vi "Get TargetRoot.vi"(8 "error in (no error)":errorcluster, 11 "Installation Directory":path) -> (0 "error out":errorcluster, 1 "Target Root Name":string, 2 "Relative Path":path)   [LabVIEW 2019, in "NIPKG Packager.lvclass"]
doc: "Calculates the Target Root directory for the NIPM Package. This is a fairly long list of potential root directories, but only a subset of common directories are handled here. This might mean in some circumstances the returned relative path is longer that if a larger collection of target roots were considered."
uses:
  NIPKG Packager.lvclass
  <vilib>/Utility/sysdir.llb/System Directory Type.ctl
  <vilib>/Utility/error.llb/Error Cluster From Error Code.vi
  <vilib>/ErrorRing/Error Ring.xnode
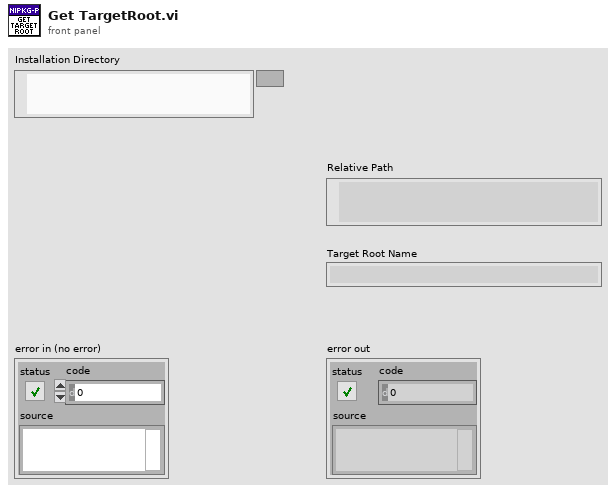
[diagram p1: front panel]
types:
  T1 = typedef "System Directory Type.ctl" = i32
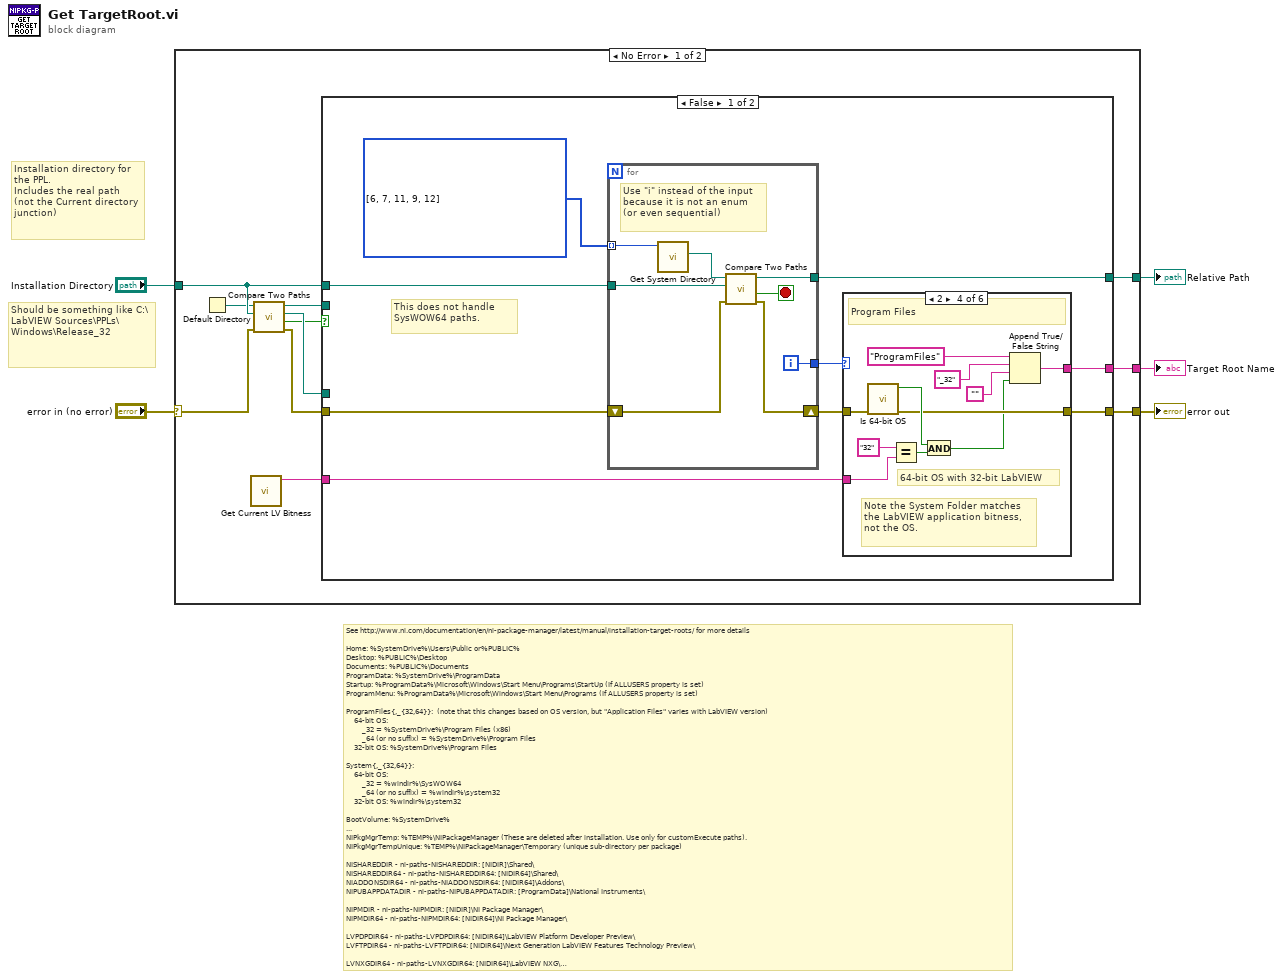
[diagram p0: block diagram]
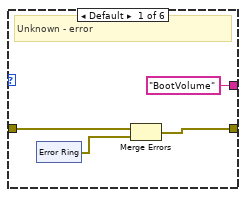
[diagram p2: hidden frame]
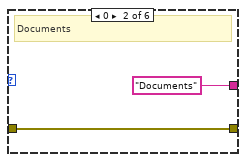
[diagram p3: hidden frame]
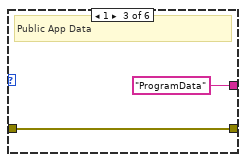
[diagram p4: hidden frame]
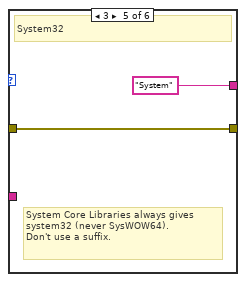
[diagram p5: hidden frame]
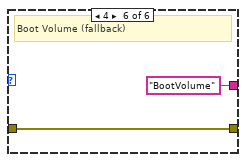
[diagram p6: hidden frame]
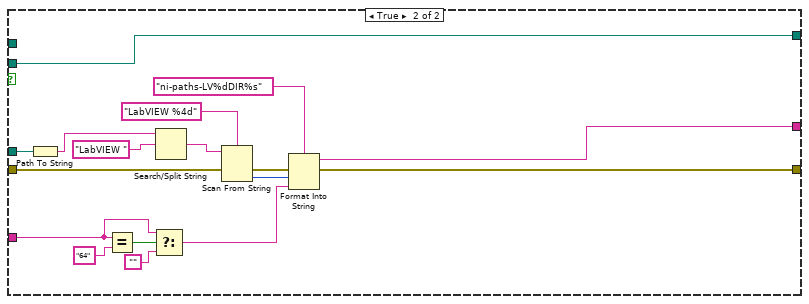
[diagram p7: hidden frame]
diagram:
  # "Should be something like C:\\LabVIEW Sources\\PPLs\\Windows\\Release_32"
  # "See http://www.ni.com/documentation/en/ni-package-manager/latest/manual/installation-target-roots/ for more details\n\nHome: %SystemDrive%\\Users\\Public or%PUBLIC%\nDesktop:\t%PUBLIC%\\Desktop\nDocuments:\t%PUBLIC%\\Documents\nProgramData: %SystemDrive%\\ProgramData\nStartup:\t%ProgramData%\\Microsoft\\Windows\\Start Menu\\Programs\\StartUp (If ALLUSERS property is set)\nProgramMenu:\t%ProgramData%\\Microsoft\\Windows\\Start Menu\\Programs (If ALLUSERS property is set)\n\nProgramFiles{,_{32,64}}:  (note that this changes based on OS version, but \"Application Files\" varies with LabVIEW version)\n    64-bit OS: \n        _32 = %SystemDrive%\\Program Files (x86)\n        _64 (or no suffix) = %SystemDrive%\\Program Files\n    32-bit OS: %SystemDrive%\\Program Files\n\nSystem{,_{32,64}}:\n    64-bit OS:\n        _32 = %windir%\\SysWOW64\n        _64 (or no suffix) = %windir%\\system32\n    32-bit OS: %windir%\\system32\n\nBootVolume:\t%SystemDrive%\n...\nNIPkgMgrTemp: %TEMP%\\NIPackageManager (These are deleted after installation. Use only for customExecute paths).\nNIPkgMgrTempUnique:\t%TEMP%\\NIPackageManager\\Temporary (unique sub-directory per package)\n\nNISHAREDDIR\t- ni-paths-NISHAREDDIR:\t[NIDIR]\\Shared\\\nNISHAREDDIR64 -\tni-paths-NISHAREDDIR64:\t[NIDIR64]\\Shared\\\nNIADDONSDIR64 -\tni-paths-NIADDONSDIR64:\t[NIDIR64]\\Addons\\\nNIPUBAPPDATADIR\t- ni-paths-NIPUBAPPDATADIR:\t[ProgramData]\\National Instruments\\\n\nNIPMDIR\t- ni-paths-NIPMDIR:\t[NIDIR]\\NI Package Manager\\\nNIPMDIR64 -\tni-paths-NIPMDIR64:\t[NIDIR64]\\NI Package Manager\\\n\nLVPDPDIR64 -\tni-paths-LVPDPDIR64:\t[NIDIR64]\\LabVIEW Platform Developer Preview\\\nLVFTPDIR64 -\tni-paths-LVFTPDIR64:\t[NIDIR64]\\Next Generation LabVIEW Features Technology Preview\\\n\nLVNXGDIR64 - ni-paths-LVNXGDIR64: [NIDIR64]\\LabVIEW NXG\\\nLVNXG200DIR64 - ni-paths-LVNXG200DIR64: [NIDIR64]\\LabVIEW NXG 2.0\\\nLVNXG300DIR64 - ni-paths-LVNXG300DIR64: [NIDIR64]\\LabVIEW NXG 3.0\\\nLVNXG400DIR64 - ni-paths-LVNXG400DIR64: [NIDIR64]\\LabVIEW NXG 4.0\\\n\nLV2014DIR - ni-paths-LV2014DIR: [NIDIR]\\LabVIEW 2014\nLV2015DIR - ni-paths-LV2015DIR: [NIDIR]\\LabVIEW 2015\nLV2016DIR - ni-paths-LV2016DIR: [NIDIR]\\LabVIEW 2016\nLV2017DIR - ni-paths-LV2017DIR: [NIDIR]\\LabVIEW 2017\nLV2018DIR - ni-paths-LV2018DIR: [NIDIR]\\LabVIEW 2018\nLV2019DIR - ni-paths-LV2019DIR: [NIDIR]\\LabVIEW 2019\n\nLV2014DIR64 - ni-paths-LV2014DIR64: [NIDIR64]\\LabVIEW 2014\nLV2015DIR64 - ni-paths-LV2015DIR64: [NIDIR64]\\LabVIEW 2015\nLV2016DIR64 - ni-paths-LV2016DIR64: [NIDIR64]\\LabVIEW 2016\nLV2017DIR64 - ni-paths-LV2017DIR64: [NIDIR64]\\LabVIEW 2017\nLV2018DIR64 - ni-paths-LV2018DIR64: [NIDIR64]\\LabVIEW 2018\nLV2019DIR64 - ni-paths-LV2019DIR64: [NIDIR64]\\LabVIEW 2019\n\nNILMLICENSESDIR\t- ni-paths-NILMLICENSESDIR:\t[NIPUBAPPDATADIR]\\License Manager\\Licenses\\\nNILMPRODUCTINFODIR\t- ni-paths-NILMPRODUCTINFODIR:\t[NIPUBAPPDATADIR]\\License Manager\\ProductInfo\\\nNILEGALROOTDIR\t- ni-paths-NILEGALROOTDIR:\t[NIDIR]\\\n\nTESTSTAND2017DIR - ni-paths-TESTSTAND2017DIR: [NIDIR]\\TestStand 2017\\\nTESTSTAND2017DIR64 - ni-paths-TESTSTAND2017DIR64: [NIDIR64]\\TestStand 2017\\\nTESTSTAND2019DIR - ni-paths-TESTSTAND2019DIR: [NIDIR]\\TestStand 2019\\\nTESTSTAND2019DIR64 - ni-paths-TESTSTAND2019DIR64: [NIDIR64]\\TestStand 2019\\\n\nNIFPGA51DIR64\t- ni-paths-NIFPGA51DIR64:\t[BootVolume]\\NIFPGA\\\n\nIVISTANDARDROOTDIR - ni-paths-IVISTANDARDROOTDIR: [Program Files_32]\\IVI Foundation\\IVI\\\nIVISTANDARDROOTDIR64 - ni-paths-IVISTANDARDROOTDIR64: [ProgramFiles_64]\\IVI Foundation\\IVI\\\nNIHELPVIEWERDOCUMENTATIONDIR\t- ni-paths-NIHELPVIEWERDOCUMENTATIONDIR:\t[NIDIR]\\Help Viewer\\Documentation\\\nMSTUDIODIR\t- ni-paths-MSTUDIODIR:\t[NIDIR]\\Measurement Studio\\"
  # "Installation directory for the PPL.\nIncludes the real path (not the Current directory junction)"
  n1 = case shown="No Error" "error in (no error)" {
    selector: "error in (no error)" -> [w13 w78]
    tunnel: [w15 w78] -> w5
    tunnel: [w14 _] -> w4
    tunnel: "Installation Directory" -> [w11 _]
    tunnel: [w6 _] -> w1
    frame No Error {
      n2 = Default Directory() -> (w10:path)
      n3 = call <vilib>:"Get Current LV Bitness.vi"() -> ("bitness"=w7:string)  [unwired: 11 in]
      n4 = call <vilib>:"Compare Two Paths.vi"("error in (no error)"=w13, "Path 2"=w11, "Path 1"=w10) -> ("error out"=w12:errorcluster, "Path 2 Relative to Path 1?"=w9:bool, "Common Path"=w16:path, "Relative Path from 1 to 2"=w8:path)  [unwired: 5 in]
      n5 = case shown="False" w9 {
        tunnel: [w19 w70] -> w15
        tunnel: [w25 w77] -> w14
        tunnel: w12 -> [w23 w66]
        tunnel: w11 -> [w22 _]
        tunnel: w8 -> [_ w77]
        tunnel: w7 -> [w17 w74]
        tunnel: w16 -> [_ w69]
        tunnel: [w18 w61] -> w6
        frame False {
          w24 = T1[] [6, 7, 11, 9, 12] items=["User Home"=0, "User Desktop"=1, "User Documents"=2, "User Application Data"=3, "User Preferences"=4, "User Temporary"=5, "Public Documents"=6, "Public Application Data"=7, "Public Preferences"=8, "Public Cache"=13, "System Core Libraries"=9, "System Installed Libraries"=10, "Application Files"=11, "Boot Volume Root"=12] ("Array")
          # "This does not handle SysWOW64 paths."
          n6 = for {
            tunnel: [w30] -> w25
            shift-right: [w31] -> w20
            shift-left: w23 -> [w32]
            tunnel: w24 -> [w27] mode=indexing
            tunnel: w22 -> [w33]
            tunnel: [w26] -> w21
            i -> [w26]
            stop <- w28 stop-if-true
            # "Use \"i\" instead of the input because it is not an enum (or even sequential)"
            n7 = call <vilib>:"Get System Directory.vi"("system directory type"=w27) -> ("system directory"=w29:path)  [unwired: 10 in]
            n8 = call <vilib>:"Compare Two Paths.vi"("error in (no error)"=w32, "Path 2"=w33, "Path 1"=w29) -> ("error out"=w31:errorcluster, "Path 2 Relative to Path 1?"=w28:bool, "Relative Path from 1 to 2"=w30:path)  [unwired: 5 in, 1 out]
          }
          n9 = case shown="2" w21 {
            tunnel: w20 -> [w37 w43 w45 w56 w58 w60]
            tunnel: [w35 w43 w45 w51 w58 w60] -> w19
            tunnel: ["BootVolume" ("output string") "Documents" "ProgramData" w50 "System" "BootVolume" ("output string")] -> w18
            tunnel: w17 -> [_ _ _ w55 _ _]
            frame Default {
              # "Unknown - error"
              n10 = xnode "Error Ring"() -> ("error out"=w34:errorcluster)
              n11 = Merge Errors(w37, w34) -> (w35:errorcluster)
            }
            frame 0 {
              # "Documents"
            }
            frame 1 {
              # "Public App Data"
            }
            frame 2 {
              # "64-bit OS with 32-bit LabVIEW"
              # "Note the System Folder matches the LabVIEW application bitness, not the OS."
              # "Program Files"
              n12 = call "Is 64-bit OS"("error in (no error)"=w56) -> ("error out"=w51:errorcluster, "64-bit OS?"=w52:bool)  [unwired: 9 in]
              n13 = Equal?(x="32", y=w55) -> (x = y?=w53:bool)
              n14 = And(x=w52, y=w53) -> (x .and. y?=w49:bool)
              n15 = Append True/False String(1:w49, 2:"", 3:"_32" ("true string"), 4:"ProgramFiles" ("string (\"\")")) -> (0:w50:string)
            }
            frame 3 {
              # "System Core Libraries always gives system32 (never SysWOW64).\nDon't use a suffix."
              # "System32"
            }
            frame 4 {
              # "Boot Volume (fallback)"
            }
          }
        }
        frame True {
          n16 = Path To String(path=w69) -> (string=w63:string)
          n17 = Equal?(x=w74, y="64") -> (x = y?=w75:bool)
          n18 = Select(t=w74, s=w75, f="") -> (s? t:f=w72:string)
          n19 = Search/Split String(string=w63, search string/char (-)="LabVIEW ") -> (match + rest of string=w62:string)  [unwired: 1 in, 2 out]
          n20 = Scan From String(format string="LabVIEW %4d", input string=w62, error in=w66) -> (error out=w67:errorcluster, output 1=w65:i32)  [unwired: 2 in, 2 out]
          n21 = Format Into String(format string="ni-paths-LV%dDIR%s", error in=w67, w65, w72) -> (resulting string=w61:string, error out=w70:errorcluster)  [unwired: 1 in]
        }
      }
    }
    frame Error {
    }
  }
  "error out" <- w5
  "Relative Path" <- w4
  "Target Root Name" <- w1
